vi "Read Test Info.vi"(8 "error in (no error)":errorcluster) -> ()   [LabVIEW 2017]
uses:
  <vilib>/Utility/config.llb/Read Key (String).vi
  SubVI - Global.vi
  <vilib>/Utility/config.llb/NI_LVConfig.lvlib
panel:
  out "Array":string[](array[string])
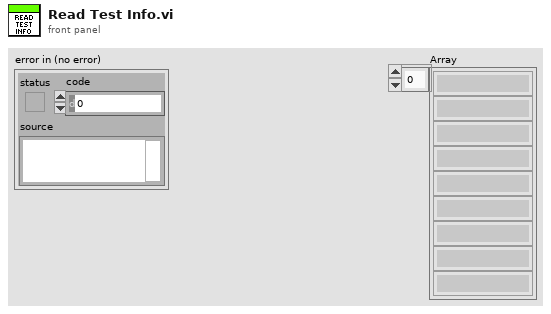
[diagram p1: front panel]
types:
  T1 = typedef "NI_LVConfig.lvlib/Config Data RefNum.ctl" = refnum<k1>
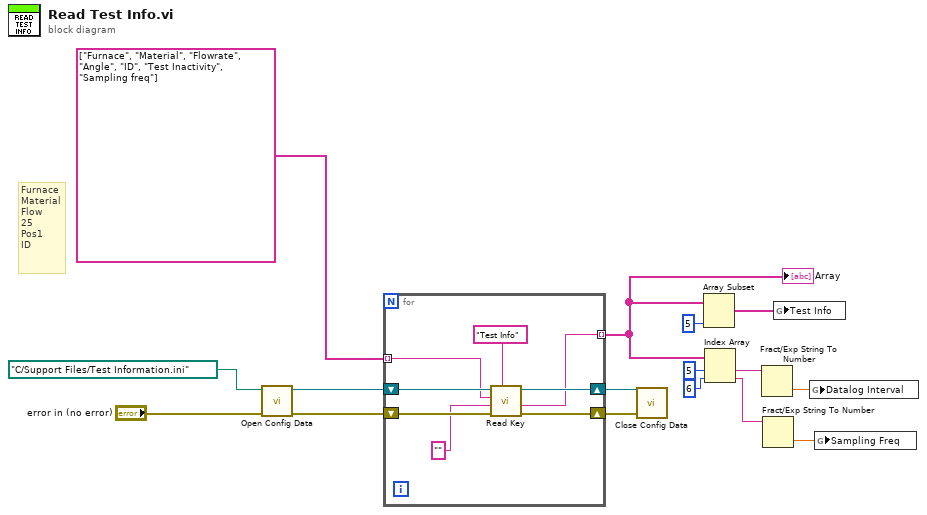
[diagram p0: block diagram]
diagram:
  # "Furnace\nMaterial\nFlow\n25\nPos1\nID"
  n1 = call <vilib>:"Open Config Data.vi"("error in (no error)"="error in (no error)", "configuration file path"=path "C:/Support Files/Test Information.ini") -> ("error out"=w14:errorcluster, "refnum"=w16:T1)  [unwired: 7 in, 1 out]
  n2 = for {
    shift-right: [w23] -> w15
    shift-left: w16 -> [w24]
    shift-right: [w21] -> w13
    shift-left: w14 -> [w22]
    tunnel: string[] ["Furnace", "Material", "Flowrate", "Angle", "ID", "Test Inactivity", "Sampling freq"] ("key") -> [w20] mode=indexing
    tunnel: [w17] -> w9 mode=indexing
    n3 = call-poly <vilib>:"Read Key.vi"("section"="Test Info", "error in (no error)"=w22, "default value"="", "key"=w20, "refnum"=w24) -> ("error out"=w21:errorcluster, "value"=w17:string, "refnum out"=w23:T1)  [unwired: 3 in, 1 out]
  }
  "Array" <- w9
  n4 = call <vilib>:"Close Config Data.vi"("error in (no error)"=w13, "refnum"=w15) -> ()  [unwired: 8 in, 2 out]
  n5 = Array Subset(array=w9, length=5) -> (w10:string[])  [unwired: 1 in]
  n6 = Index Array(array=w9, index #1=5 ("index"), index #2=6 ("index")) -> (element #1=w7:string, element #2=w1:string)
  n7 = Fract/Exp String To Number(string=w7) -> (number=w6:dbl)  [unwired: 3 in, 1 out]
  n8 = Fract/Exp String To Number(string=w1) -> (number=w4:dbl)  [unwired: 3 in, 1 out]
  n9 = global write "SubVI - Global.vi" "Test Info"(w10) -> ()
  n10 = global write "SubVI - Global.vi" "Datalog Interval"(w6) -> ()
  n11 = global write "SubVI - Global.vi" "Sampling Freq"(w4) -> ()
